vi "7pt Mov Avg.vi"(10 "Value in":dbl) -> (2 "Value out":dbl)   [LabVIEW 2014]
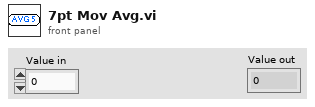
[diagram p1: front panel]
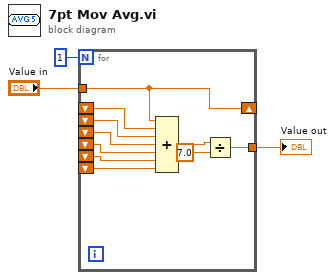
[diagram p0: block diagram]
diagram:
  n1 = for {
    N: 1 -> [_]
    tunnel: "Value in" -> [w13]
    shift-right: [w13] -> _
    shift-left: _ -> [w12]
    shift-left: _ -> [w11]
    tunnel: [w8] -> w1
    shift-left: _ -> [w7]
    shift-left: _ -> [w6]
    shift-left: _ -> [w5]
    shift-left: _ -> [w4]
    n2 = Compound Arithmetic op=ADD(w13, w12, w11, w7, w6, w5, w4) -> (w10:dbl)
    n3 = Divide(x=w10, y=7.0) -> (x/y=w8:dbl)
  }
  "Value out" <- w1
